vi "Load Calibration from text file.vi"(7 "path":string, 8 "error in (no error)":errorcluster, 11 "PathControl in":refnum<class "PathControl.lvclass">) -> (0 "error out":errorcluster, 3 "PathControl out":refnum<class "PathControl.lvclass">)   [LabVIEW 2020, in "PathControl.lvclass"]
uses:
  PathControl.lvclass
  Measurements Specific Paths.ctl
  Paths.ctl
panel:
  out "XY Graph":cluster{dbl[], dbl[]}(graph)
  out "Path":T1
  out "Measurement specfic paths":T2
  in  "Cancel Button":bool
  in  "OK Button":bool
  in  "File Path":path
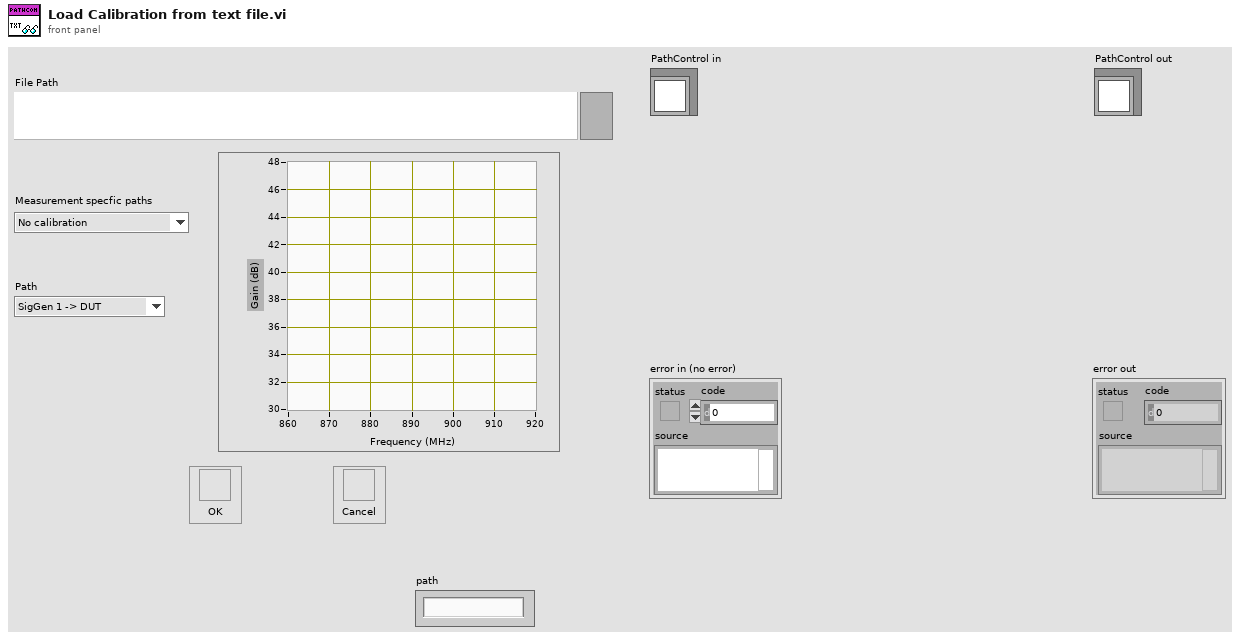
[diagram p1: front panel]
types:
  T1 = typedef "PathControl.lvclass/Paths.ctl" = enum16{"SigGen 1 -> DUT", "SigGen 2 -> DUT", "SigGen 1 -> PM 1", "SigGen 1 -> PM 2", "DUT -> SA", "DUT -> PM 2", "VSG -> DUT", "SigGen 2 -> PM 1", "SigGen 2 -> PM 2"}
  T2 = typedef "PathControl.lvclass/Measurements Specific Paths.ctl" = enum16{"No calibration", "Harmonics", "IMD", "S Parameter", "AM-AM", "MCCW-ACLR", "DC", "LCR", "Power Meter GUI", "RF Power"}
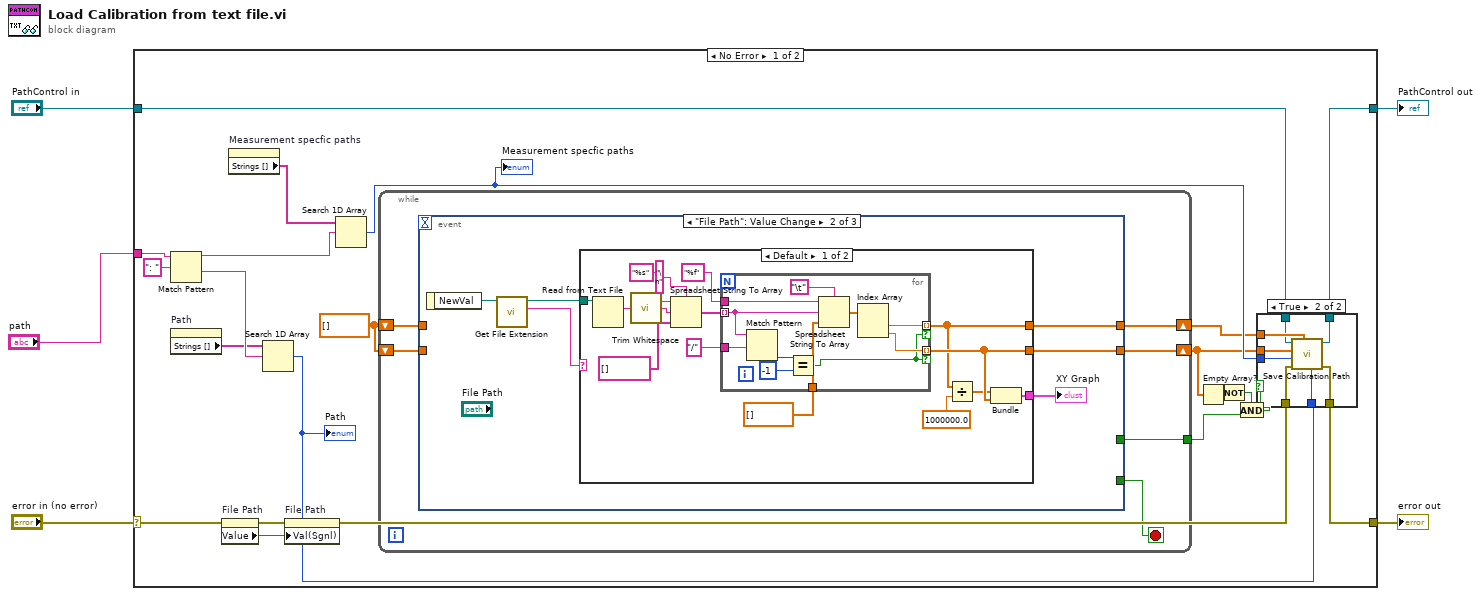
[diagram p0: block diagram]
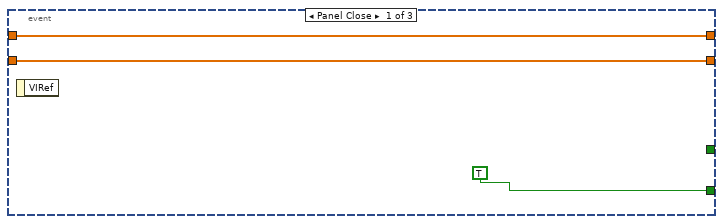
[diagram p3: hidden frame]
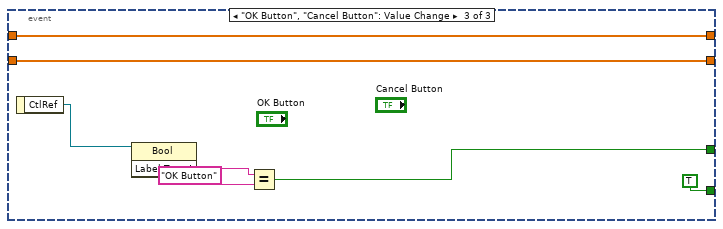
[diagram p5: hidden frame]
diagram:
  n1 = case shown="No Error" "error in (no error)" {
    selector: "error in (no error)" -> [w6 w87]
    tunnel: [w19 w87] -> w4
    tunnel: [w20 w86] -> w2
    tunnel: "PathControl in" -> [w21 w86]
    tunnel: "path" -> [w24 _]
    frame No Error {
      w15 = dbl[] []
      n2 = Match Pattern(string=w24, regular expression=": ") -> (before substring=w26:string, after substring=w27:string)  [unwired: 1 in, 2 out]
      n3 = property on="Path" class="Enum (strict)"() -> ("Strings []"=w23:string[])  [unwired: 2 in, 2 out]
      n4 = property on="File Path" class="Path"(error in=w6) -> (error out=w7:errorcluster, "Value"=w8:path)  [unwired: 1 in, 1 out]
      n5 = property on="Measurement specfic paths" class="Enum (strict)"() -> ("Strings []"=w22:string[])  [unwired: 2 in, 2 out]
      n6 = Search 1D Array(1D array=w23, element=w27) -> (index of element=w17:i32)  [unwired: 1 in]
      "Path" <- w17
      n7 = property on="File Path" class="Path"(error in=w7, "Val(Sgnl)"=w8) -> (error out=w9:errorcluster)  [unwired: 1 in, 1 out]
      n8 = Search 1D Array(1D array=w22, element=w26) -> (index of element=w18:i32)  [unwired: 1 in]
      "Measurement specfic paths" <- w18
      n9 = while {
        shift-right: [w42] -> w16
        shift-left: w15 -> [w39]
        shift-right: [w41] -> w12
        shift-left: w15 -> [w40]
        tunnel: [w38] -> w11
        stop <- w43 stop-if-true
        n10 = event shown="[1] \"File Path\": Value Change" {
          selector: _ -> [_ _ _]
          dyn-events: _ -> [_ _ _]
          timeout: _ -> [_ _ _]
          tunnel: [TRUE _ TRUE] -> w43
          tunnel: [w44 w49 w80] -> w42
          tunnel: [w45 w48 w81] -> w41
          tunnel: w40 -> [w45 _ w81]
          tunnel: w39 -> [w44 _ w80]
          tunnel: [_ _ w82] -> w38
          event Panel Close {
            n11 = event-data() -> ()  [unwired: 1 in, 1 out]
          }
          event "File Path": Value Change {
            n12 = event-data() -> ("NewVal"=w52:path)  [unwired: 1 in]
            n13 = call <vilib>:"Get File Extension.vi"("file"=w52) -> ("lowercase file extension"=w51:string, "dup file"=w50:path)  [unwired: 6 in, 3 out]
            n14 = case shown="Default" w51 {
              tunnel: w50 -> [w67 _]
              tunnel: [w56 _] -> w49
              tunnel: [w60 _] -> w48
              tunnel: [w54 _] -> w47
              frame Default {
                n15 = Read from Text File(file (use dialog)=w67) -> (text=w59:string)  [unwired: 3 in, 3 out]
                n16 = call <vilib>:"Trim Whitespace.vi"("string"=w59) -> ("trimmed string"=w58:string)  [unwired: 1 in]
                n17 = Spreadsheet String To Array(delimiter (Tab)="\n", format string="%s", spreadsheet string=w58, array type (2D Dbl)=string[] []) -> (array=w66:string[])
                n18 = for {
                  tunnel: w66 -> [w73] mode=indexing
                  tunnel: "%f" -> [w78]
                  tunnel: [w76] -> w56 mode=indexing if=w70
                  tunnel: [w75] -> w60 mode=indexing if=w70
                  tunnel: dbl[] [] -> [w74]
                  tunnel: "/" ("delimiter (Tab)") -> [w68]
                  n19 = Match Pattern(string=w73, regular expression=w68) -> (offset past match=w72:i32)  [unwired: 1 in, 3 out]
                  n20 = Equal?(x=w72, y=-1) -> (x = y?=w70:bool)
                  n21 = Spreadsheet String To Array(delimiter (Tab)="\t", format string=w78, spreadsheet string=w73, array type (2D Dbl)=w74) -> (array=w77:dbl[])
                  n22 = Index Array(array=w77) -> (element #1=w76:dbl, element #2=w75:dbl)  [unwired: 2 in]
                }
                n23 = Divide(x=w56, y=1000000.0) -> (x/y=w55:dbl[])
                n24 = Bundle(w55, w60) -> (w54:cluster{dbl[], dbl[]})  [unwired: 1 in]
              }
              frame "xml" {
                # "Future support"
              }
            }
            "XY Graph" <- w47
          }
          event "OK Button", "Cancel Button": Value Change {
            n25 = event-data() -> ("CtlRef"=w83:refnum<vi>)  [unwired: 1 in]
            n26 = property class="Bool"(reference=w83) -> ("Label.Text"=w85:string)  [unwired: 1 in, 2 out]
            n27 = Equal?(x=w85, y="OK Button") -> (x = y?=w82:bool)
          }
        }
      }
      n28 = Empty Array?(array=w12) -> (empty?=w14:bool)
      n29 = Not(x=w14) -> (.not. x?=w13:bool)
      n30 = And(x=w13, y=w11) -> (x .and. y?=w10:bool)
      n31 = case shown="True" w10 {
        tunnel: w16 -> [_ w37]
        tunnel: w21 -> [w28 w36]
        tunnel: [w28 w35] -> w20
        tunnel: w12 -> [_ w34]
        tunnel: w18 -> [_ w33]
        tunnel: w17 -> [_ w32]
        tunnel: w9 -> [w29 w31]
        tunnel: [w29 w30] -> w19
        frame False {
        }
        frame True {
          n32 = call "Save Calibration Path.vi"("Path"=w32, "Frequency"=w37, "Error In"=w31, "Measurement specfic paths"=w33, "Path Loss"=w34, "PathControl in"=w36) -> ("Error Out"=w30:errorcluster, "PathControl out"=w35:refnum<class "PathControl.lvclass">)  [unwired: 4 in]
        }
      }
    }
    frame Error {
    }
  }
  "error out" <- w4
  "PathControl out" <- w2
